vi "Open.vi"(8 "error in (no error)":errorcluster, 11 "PowerSupplyVisa in":refnum<class "PowerSupplyVisa.lvclass">) -> (0 "error out":errorcluster, 3 "PowerSupplyVisa out":refnum<class "PowerSupplyVisa.lvclass">)   [LabVIEW 2020, in "LAF2024Q2.lvlib" / "PowerSupplyVisa.lvclass"]
uses:
  PowerSupplyVisa.lvclass
  PowerSupplyVisa.lvclass/PowerSupplyVisa.ctl
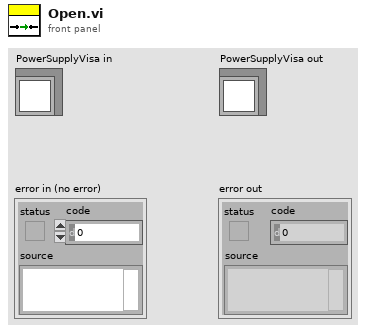
[diagram p1: front panel]
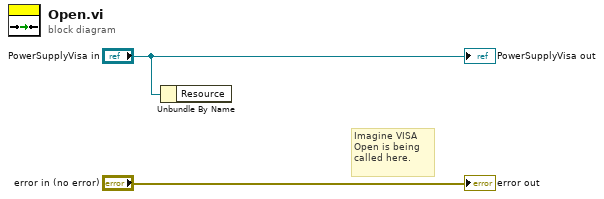
[diagram p0: block diagram]
diagram:
  # "Imagine VISA Open is being called here."
  n1 = Unbundle By Name("PowerSupplyVisa in") -> ()  [unwired: 1 out]
  "error out" <- "error in (no error)"
  "PowerSupplyVisa out" <- "PowerSupplyVisa in"
